vi "Configure Date.vi"(8 "error in (no error)":errorcluster, 10 "Time Stamp":timestamp=timestamp(3512061313.5513387 s since 1904-01-01), 11 "VISA resource name":refnum<visa-resource-name>) -> (0 "error out":errorcluster, 3 "VISA resource name out":refnum<visa-resource-name>)   [LabVIEW 2015, in "BK Precision 983X Series.lvlib"]
doc: "Configure the instrument's system time and date."
uses:
  <instrlib>/BK Precision 983X Series/BK Precision 983X Series.lvlib
  <vilib>/regexp/Match Regular Expression.xnode
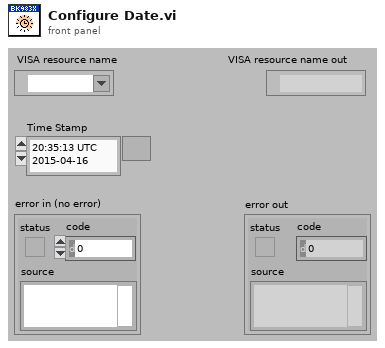
[diagram p1: front panel]
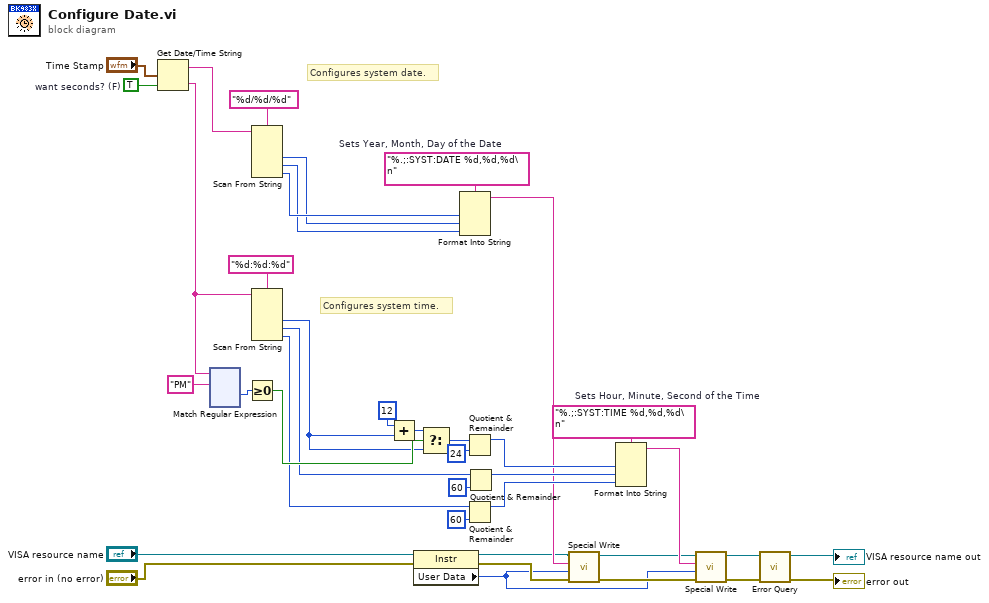
[diagram p0: block diagram]
diagram:
  w27 = "%.;:SYST:TIME %d,%d,%d\n"  # Sets Hour, Minute, Second of the Time
  w37 = TRUE  # want seconds? (F)
  w39 = "%.;:SYST:DATE %d,%d,%d\n"  # Sets Year, Month, Day of the Date
  # "Configures system time."
  # "Configures system date."
  n1 = Get Date/Time String(seconds (now)="Time Stamp", want seconds? (F)=w37) -> (date string=w35:string, time string=w19:string)  [unwired: 1 in]
  n2 = xnode ("Match Regular Expression")("input string"=w19, "regular expression"="PM" ("format string")) -> ("offset past match"=w17:i32)  [unwired: 4 in, 4 out]
  n3 = Greater Or Equal To 0?(x=w17) -> (x >= 0?=w33:bool)
  n4 = Scan From String(format string="%d/%d/%d", input string=w35) -> (output 1=w15:i32, output 2=w14:i32, output 3=w16:i32)  [unwired: 5 in, 3 out]
  n5 = Scan From String(format string="%d:%d:%d", input string=w19) -> (output 1=w32:i32, output 2=w25:i32, output 3=w21:i32)  [unwired: 5 in, 3 out]
  n6 = Add(x=12, y=w32) -> (x+y=w30:i32)
  n7 = property on="Property Node" class="Instr"(reference="VISA resource name", error in="error in (no error)") -> (reference out=w3:refnum<visa-resource-name>, error out=w2:errorcluster, "User Data"=w1:u32)
  n8 = Select(t=w30, s=w33, f=w32) -> (s? t:f=w29:i32)
  n9 = Format Into String(format string=w39, w16, w15, w14) -> (resulting string=w4:string)  [unwired: 2 in, 1 out]
  n10 = Quotient & Remainder(x=w29, y=24) -> (x-y*floor(x/y)=w26:i32)  [unwired: 1 out]
  n11 = Quotient & Remainder(x=w21, y=60) -> (x-y*floor(x/y)=w20:i32)  [unwired: 1 out]
  n12 = Quotient & Remainder(x=w25, y=60) -> (x-y*floor(x/y)=w23:i32)  [unwired: 1 out]
  n13 = call <instrlib>:"Special Write.vi"("error in (no error)"=w2, "Delay (0 ms)"=w1, "Input String"=w4, "VISA resource name"=w3) -> ("error out"=w5:errorcluster, "VISA resource name out"=w6:refnum<visa-resource-name>)  [unwired: 6 in]
  n14 = Format Into String(format string=w27, w26, w23, w20) -> (resulting string=w7:string)  [unwired: 2 in, 1 out]
  n15 = call <instrlib>:"Special Write.vi"("error in (no error)"=w5, "Delay (0 ms)"=w1, "Input String"=w7, "VISA resource name"=w6) -> ("error out"=w8:errorcluster, "VISA resource name out"=w11:refnum<visa-resource-name>)  [unwired: 6 in]
  n16 = call <instrlib>:"Error Query.vi"("error in (no error)"=w8, "VISA resource name"=w11) -> ("error out"=→"error out":errorcluster, "VISA resource name out"=→"VISA resource name out":refnum<visa-resource-name>)  [unwired: 6 in, 2 out]
